vi "get_line_scan_time.vi"(8 "error in (no error)":errorcluster, 11 "ImagingModeDL090130Frame in":refnum<class "ImagingModeDL090130Frame.lvclass">=refnum) -> (0 "error out":errorcluster, 2 "line-scan time":dbl[unit], 3 "ImagingModeDL090130Frame out":refnum<class "ImagingModeDL090130Frame.lvclass">)   [LabVIEW 2010, in "ImagingModeDL090130Frame.lvclass"]
uses:
  ImagingModeDL090130Frame.lvclass
  ImagingModeDL090130Frame.lvclass/ImagingModeDL090130Frame.ctl
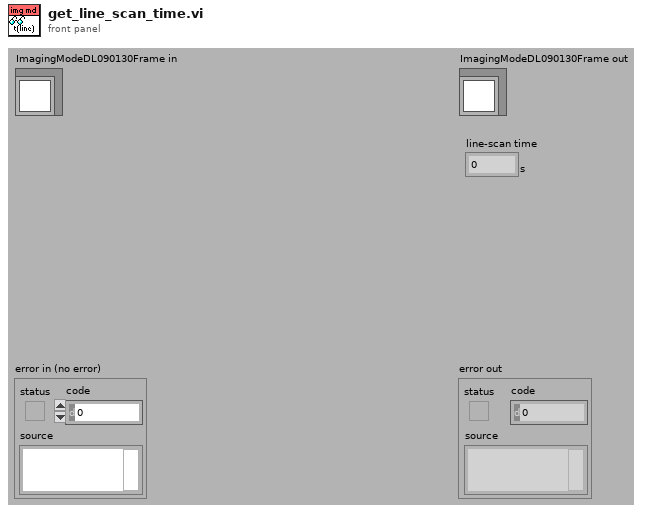
[diagram p1: front panel]
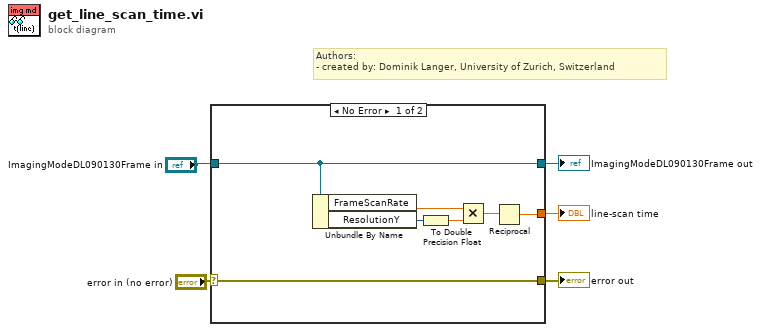
[diagram p0: block diagram]
diagram:
  # "Authors: \n- created by: Dominik Langer, University of Zurich, Switzerland"
  n1 = case shown="No Error" "error in (no error)" {
    selector: "error in (no error)" -> [w12 w14]
    tunnel: [w12 w14] -> w4
    tunnel: [w11 w13] -> w2
    tunnel: "ImagingModeDL090130Frame in" -> [w11 w13]
    tunnel: [w6 _] -> w1
    frame No Error {
      n2 = Unbundle By Name(w11) -> ("FrameScanRate"=w8:dbl[unit], "ResolutionY"=w10:i32)
      n3 = To Double Precision Float(number=w10) -> (double precision float=w9:dbl)
      n4 = Multiply(x=w8, y=w9) -> (x*y=w7:dbl[unit])
      n5 = Reciprocal(x=w7) -> (1/x=w6:dbl[unit])
    }
    frame Error {
    }
  }
  "error out" <- w4
  "ImagingModeDL090130Frame out" <- w2
  "line-scan time" <- w1
